vi "EXCOM_26.vi"(0 "VRN IN":refnum<visa-resource-name>, 11 "Error IN":errorcluster) -> (2 "STATL":bool[](array[boolean])=[TRUE, FALSE, FALSE, FALSE, FALSE, FALSE, FALSE, FALSE, FALSE, FALSE, FALSE, FALSE, FALSE, FALSE, FALSE, FALSE, FALSE, FALSE, FALSE, FALSE, FALSE, FALSE, FALSE, FALSE, FALSE, FALSE, FALSE, FALSE, FALSE, FALSE, FALSE, FALSE], 3 "STATH":bool[](array[boolean])=[FALSE, FALSE, TRUE, TRUE, FALSE, TRUE, TRUE, FALSE, FALSE, FALSE, FALSE, FALSE, FALSE, FALSE, FALSE, FALSE, FALSE, FALSE, FALSE, FALSE, FALSE, FALSE, FALSE, FALSE, FALSE, FALSE, FALSE, FALSE, FALSE, FALSE, FALSE, FALSE], 4 "VRN OUT":refnum<visa-resource-name>, 8 "OK Done":bool=TRUE, 13 "STATEX":bool[](array[boolean]), 14 "STATLH":bool[](array[boolean]), 15 "Error OUT":errorcluster)   [LabVIEW 2011]
panel:
  out "SendTime":u32
  out "SortingTime":u32
  out "Answer":string
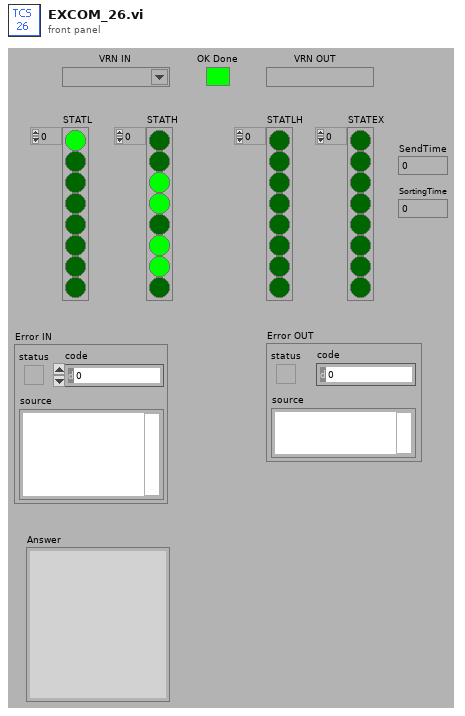
[diagram p1: front panel]
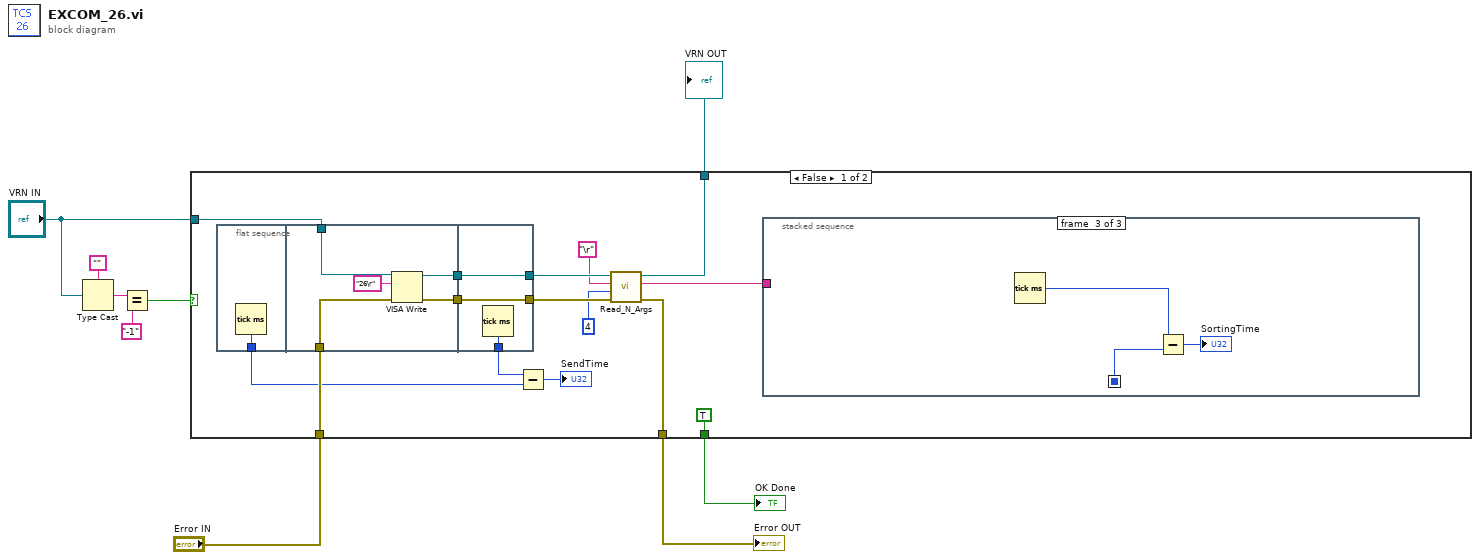
[diagram p0: block diagram]
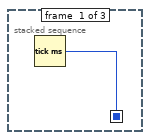
[diagram p2: hidden frame]
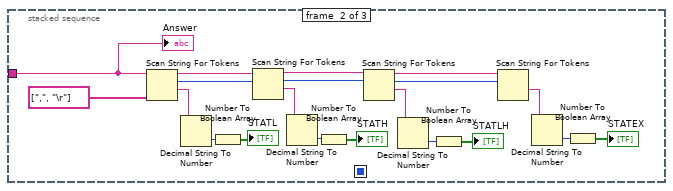
[diagram p3: hidden frame]
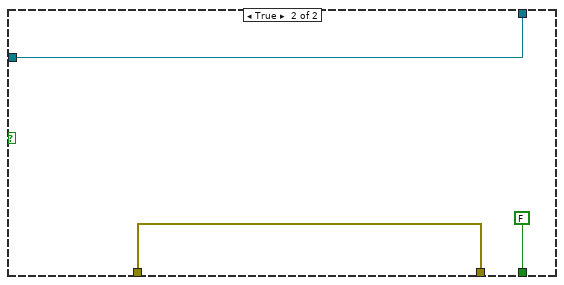
[diagram p4: hidden frame]
diagram:
  n1 = Type Cast(type="", x="VRN IN") -> (*(type *) &x=w8:string)
  n2 = Equal?(x=w8, y="-1") -> (x = y?=w5:bool)
  n3 = case shown="False" w5 {
    tunnel: "VRN IN" -> [w16 w60]
    tunnel: [w17 w60] -> w4
    tunnel: [w19 w58] -> w3
    tunnel: [TRUE ("status") FALSE ("status")] -> w2
    tunnel: "Error IN" -> [w15 w58]
    frame False {
      n4 = flat-sequence {
        tunnel: [w25] -> w11
        tunnel: w16 -> [w27]
        tunnel: w15 -> [w26]
        tunnel: [w29] -> w14
        tunnel: [w28] -> w13
        tunnel: [w32] -> w23
        tunnel: [w33] -> w24
        tunnel: w14 -> [w33]
        tunnel: w13 -> [w32]
        tunnel: [w31] -> w12
        frame #0 {
          n5 = Tick Count (ms)() -> (millisecond timer value=w25:u32)
        }
        frame #1 {
          n6 = VISA Write(VISA resource name=w27, write buffer="26\r" ("String to Send"), error in (no error)=w26) -> (VISA resource name out=w28:refnum<visa-resource-name>, error out=w29:errorcluster)  [unwired: 1 out]
        }
        frame #2 {
          n7 = Tick Count (ms)() -> (millisecond timer value=w31:u32)
        }
      }
      n8 = Subtract(x=w12, y=w11) -> (x-y=→"SendTime":u32)
      n9 = call "Read_N_Args.vi"("Error IN"=w24, "Nb_Args"=4, "Arg_Char"="\r", "VRN IN"=w23) -> ("Error OUT"=w19:errorcluster, "Answer"=w20:string, "VRN OUT"=w17:refnum<visa-resource-name>)  [unwired: 4 in, 1 out]
      n10 = stacked-sequence {
        seq-local: [w34 _ _] -> [_ _ w56]
        tunnel: w20 -> [_ w35 _]
        frame #0 {
          n11 = Tick Count (ms)() -> (millisecond timer value=w34:u32)
        }
        frame #1 {
          n12 = Scan String For Tokens(6:string[] [",", "\r"] ("delimiters (\\s,\\t,\\r,\\n)"), 9:w35) -> (1:w54:string, 2:w48:i32, 3:w50:string)  [unwired: 4 in, 1 out]
          n13 = Decimal String To Number(string=w54) -> (number=w46:i32)  [unwired: 2 in, 1 out]
          n14 = Number To Boolean Array(number=w46) -> (Boolean array=→"STATL":bool[])
          n15 = Scan String For Tokens(8:w48, 9:w50) -> (1:w52:string, 2:w47:i32, 3:w49:string)  [unwired: 4 in, 1 out]
          n16 = Decimal String To Number(string=w52) -> (number=w44:i32)  [unwired: 2 in, 1 out]
          n17 = Number To Boolean Array(number=w44) -> (Boolean array=→"STATH":bool[])
          n18 = Scan String For Tokens(8:w47, 9:w49) -> (1:w51:string, 2:w38:i32, 3:w37:string)  [unwired: 4 in, 1 out]
          n19 = Decimal String To Number(string=w51) -> (number=w43:i32)  [unwired: 2 in, 1 out]
          n20 = Number To Boolean Array(number=w43) -> (Boolean array=→"STATLH":bool[])
          n21 = Scan String For Tokens(8:w38, 9:w37) -> (1:w40:string)  [unwired: 4 in, 3 out]
          n22 = Decimal String To Number(string=w40) -> (number=w39:i32)  [unwired: 2 in, 1 out]
          n23 = Number To Boolean Array(number=w39) -> (Boolean array=→"STATEX":bool[])
          "Answer" <- w35
        }
        frame #2 {
          n24 = Tick Count (ms)() -> (millisecond timer value=w57:u32)
          n25 = Subtract(x=w57, y=w56) -> (x-y=→"SortingTime":u32)
        }
      }
    }
    frame True {
    }
  }
  "VRN OUT" <- w4
  "Error OUT" <- w3
  "OK Done" <- w2
